vi "PointMap_Update.vi"(8 "error in (no error)":errorcluster, 10 "Name":string, 11 "Map":refnum<data-value>) -> (0 "error out":errorcluster)   [LabVIEW 2017, in "PointValueMap.lvlib"]
doc: "Replaces an existing map in memory with a different map."
uses:
  <vilib>/addons/PointValueMap/PointValueMap.lvlib
  <vilib>/addons/PointValueMap/controls/PointMapOperations.ctl
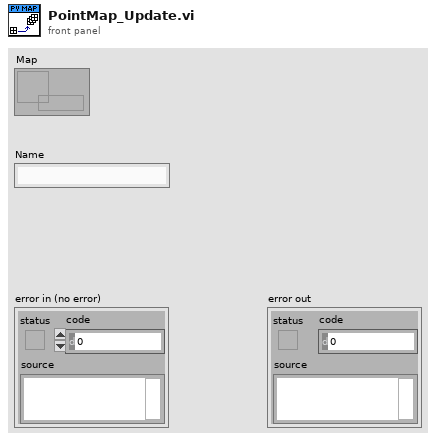
[diagram p1: front panel]
types:
  T1 = typedef "PointValueMap.lvlib/PointMapOperations.ctl" = enum16{"Initialize", "Create Map", "Update Map", "Get Map", "Get All Maps", "Destroy Map", "Destroy All Maps"}
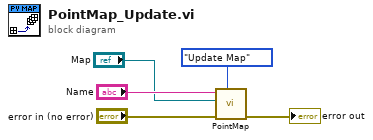
[diagram p0: block diagram]
diagram:
  n1 = call <vilib>:"PointMap.vi"("Operation"=PointMapOperations."Update Map", "error in (no error)"="error in (no error)", "Map"="Map", "Name"="Name") -> ("error out"=→"error out":errorcluster)  [unwired: 3 in, 4 out]
